vi "Enable or Disable Button.vi"(8 "Error In":errorcluster, 9 "Mark Selected Errors As Read Button Reference":refnum<vi>, 10 "MCL Value":i32[](array[numeric]), 11 "Handled Errors (MCL Display Order)":T1[](array[typedef])) -> (0 "Error Out":errorcluster)   [LabVIEW 2016, in "Error Manager.lvlib" / "Mark Selected Errors As Read Button.lvclass"]
doc: "This VI determines whether the \"Mark Selected Errors As Read\" button should be enabled or disabled and greyed out. The button should be enabled only when the user has selected one or more rows that represent unread errors."
uses:
  Mark Selected Errors As Read Button.lvclass
  Private VIs/Read-Unread Status (enum).ctl
  Error Manager.lvlib
  Private VIs/Handled Error (cluster).ctl
panel:
  out "Number of MCL rows selected":i32
  # "Development\nControls or indicators that are useful for development or testing, but which are not outputs of the VI."
  # "Input\nInputs to the VI"
  # "Output\nOutputs of the VI"
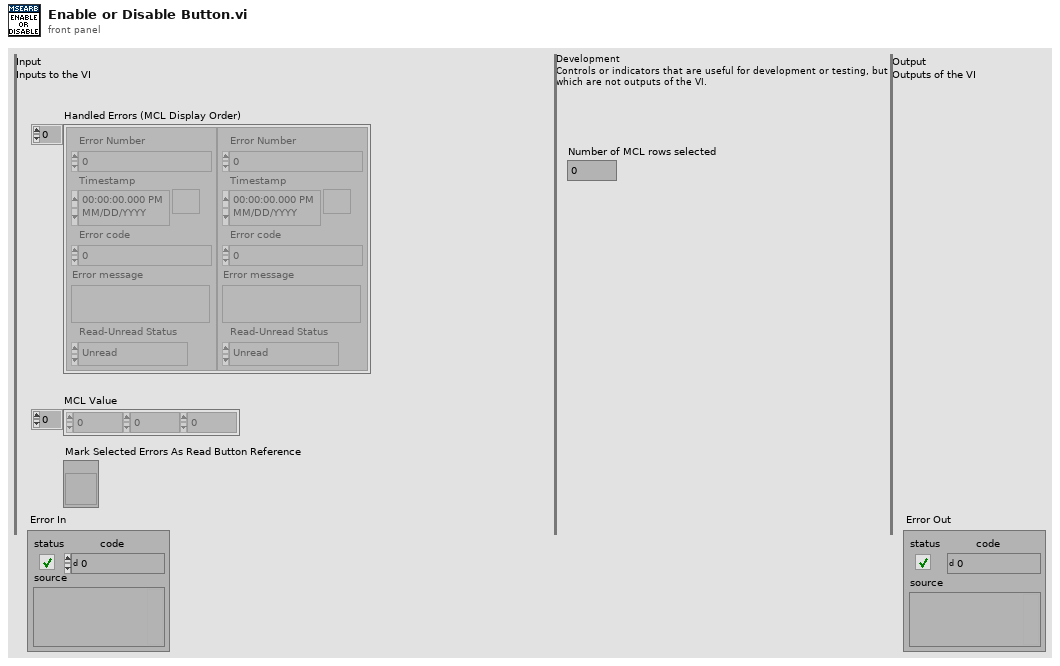
[diagram p1: front panel]
types:
  T1 = typedef "Error Manager.lvlib/Handled Error (cluster).ctl" = cluster{"Error Number":i32, "Timestamp":timestamp, "Error code":i32, "Error message":string, "Read-Unread Status":T2}
  T2 = typedef "Error Manager.lvlib/Read-Unread Status (enum).ctl" = enum16{"Unread", "Read"}
  T3 = enum8{"Enabled", "Disabled", "Disabled and Grayed Out"}
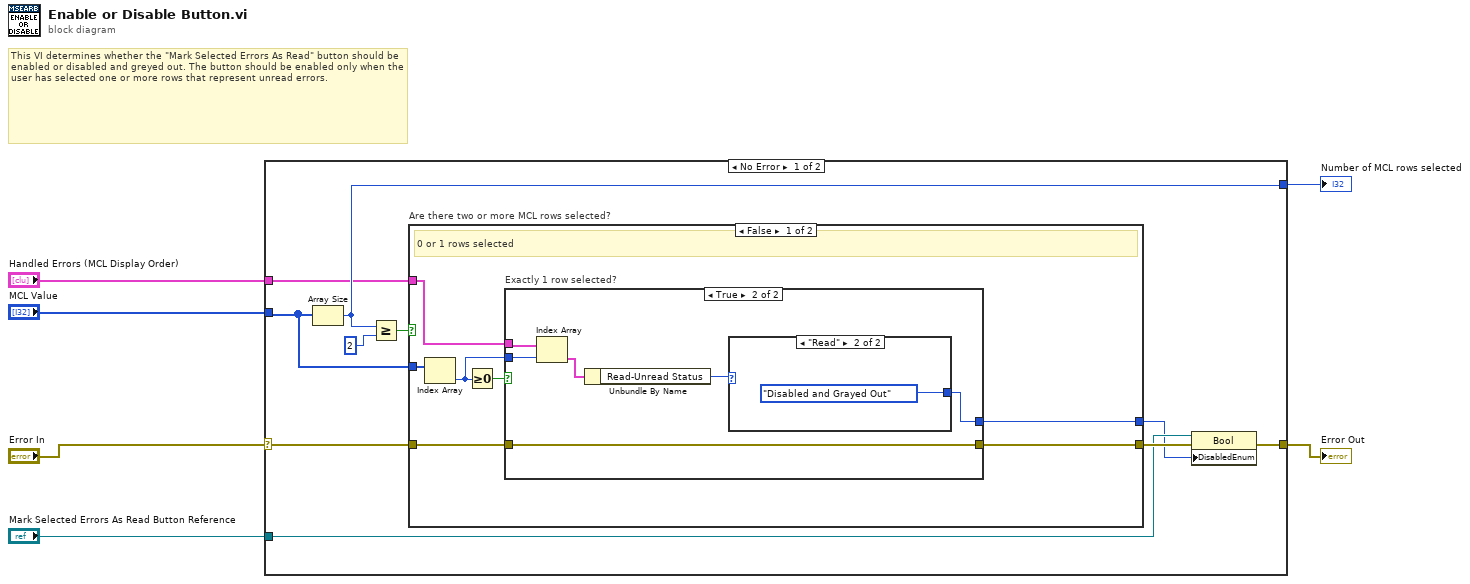
[diagram p0: block diagram]
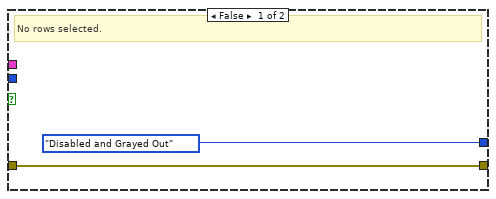
[diagram p2: hidden frame]
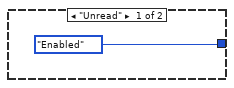
[diagram p3: hidden frame]
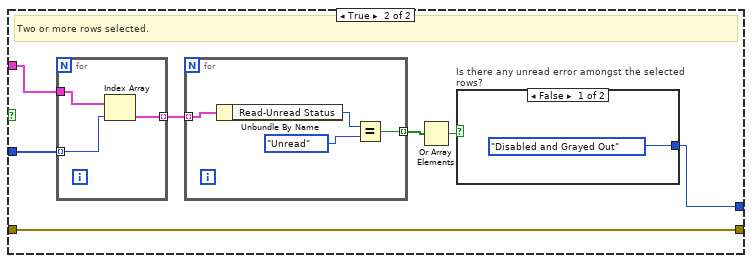
[diagram p4: hidden frame]
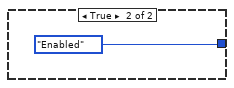
[diagram p5: hidden frame]
diagram:
  # "This VI determines whether the \"Mark Selected Errors As Read\" button should be enabled or disabled and greyed out. The button should be enabled only when the user has selected one or more rows that represent unread errors."
  n1 = case shown="No Error" "Error In" {
    selector: "Error In" -> [w16 w50]
    tunnel: [w10 w50] -> w5
    tunnel: "Handled Errors (MCL Display Order)" -> [w7 _]
    tunnel: "MCL Value" -> [w11 _]
    tunnel: [w12 _] -> w2
    tunnel: "Mark Selected Errors As Read Button Reference" -> [w9 _]
    frame No Error {
      n2 = Array Size(array=w11) -> (size(s)=w12:i32)
      n3 = Greater Or Equal?(x=w12, y=2) -> (x >= y?=w13:bool)
      n4 = case "Are there two or more MCL rows selected?" shown="False" w13 {
        tunnel: w16 -> [w23 w40]
        tunnel: [w21 w40] -> w14
        tunnel: w11 -> [w22 w38]
        tunnel: [w19 w34] -> w8
        tunnel: w7 -> [w18 w39]
        frame False {
          # "0 or 1 rows selected"
          n5 = Index Array(array=w22) -> (element=w17:i32)  [unwired: 1 in]
          n6 = Greater Or Equal To 0?(x=w17) -> (x >= 0?=w20:bool)
          n7 = case "Exactly 1 row selected?" shown="True" w20 {
            tunnel: w23 -> [w25 w31]
            tunnel: [w25 w31] -> w21
            tunnel: [T3."Disabled and Grayed Out" ("Disabled") w26] -> w19
            tunnel: w18 -> [_ w29]
            tunnel: w17 -> [_ w30]
            frame False {
              # "No rows selected."
            }
            frame True {
              n8 = Index Array(array=w29, index=w30) -> (element=w28:T1)
              n9 = Unbundle By Name(w28) -> ("Read-Unread Status"=w27:T2)
              n10 = case shown="\"Read\"" w27 {
                tunnel: [T3."Enabled" ("Disabled") T3."Disabled and Grayed Out" ("Disabled")] -> w26
                frame "Unread" {
                }
                frame "Read" {
                }
              }
            }
          }
        }
        frame True {
          # "Two or more rows selected."
          n11 = for {
            tunnel: w39 -> [w49]
            tunnel: w38 -> [w48] mode=indexing
            tunnel: [w47] -> w37 mode=indexing
            n12 = Index Array(array=w49, index=w48) -> (element=w47:T1)
          }
          n13 = for {
            tunnel: w37 -> [w46] mode=indexing
            tunnel: [w43] -> w36 mode=indexing
            n14 = Unbundle By Name(w46) -> ("Read-Unread Status"=w45:T2)
            n15 = Equal?(x=w45, y=Read-Unread_Status_(enum)."Unread") -> (x = y?=w43:bool)
          }
          n16 = Or Array Elements(Boolean array=w36) -> (logical OR=w35:bool)
          n17 = case "Is there any unread error amongst the selected rows?" shown="False" w35 {
            tunnel: [T3."Disabled and Grayed Out" ("Disabled") T3."Enabled" ("Disabled")] -> w34
            frame False {
            }
            frame True {
            }
          }
        }
      }
      n18 = property class="Bool"(reference=w9, error in=w14, "DisabledEnum"=w8) -> (error out=w10:errorcluster)  [unwired: 1 out]
    }
    frame Error {
    }
  }
  "Error Out" <- w5
  "Number of MCL rows selected" <- w2
